vi "Read.vi"(8 "error in (no error)":errorcluster, 11 "UDP Reader in":refnum<class "UDP Reader.lvclass">) -> (0 "error out":errorcluster, 3 "UDP Reader out":refnum<class "UDP Reader.lvclass">)   [LabVIEW 2022 SP3, in "UDP Reader.lvlib" / "UDP Reader.lvclass"]
uses:
  UDP Reader.lvclass
  UDP Reader.lvclass/UDP Reader.ctl
  <vilib>/event_ctls.llb/usereventprio.ctl
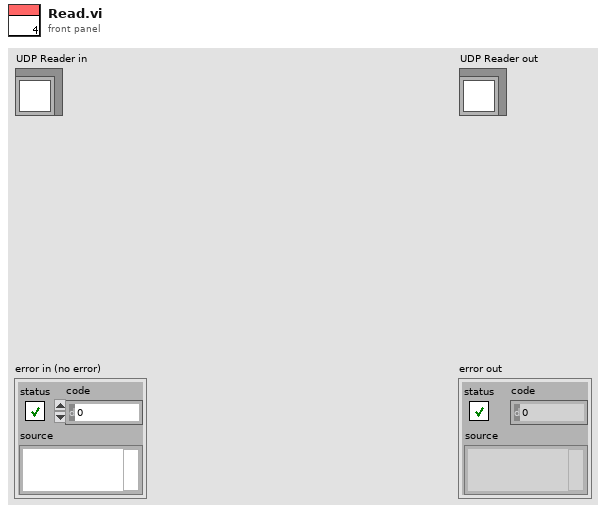
[diagram p1: front panel]
types:
  T1 = typedef "usereventprio.ctl" = enum32{"high priority", "normal priority"}
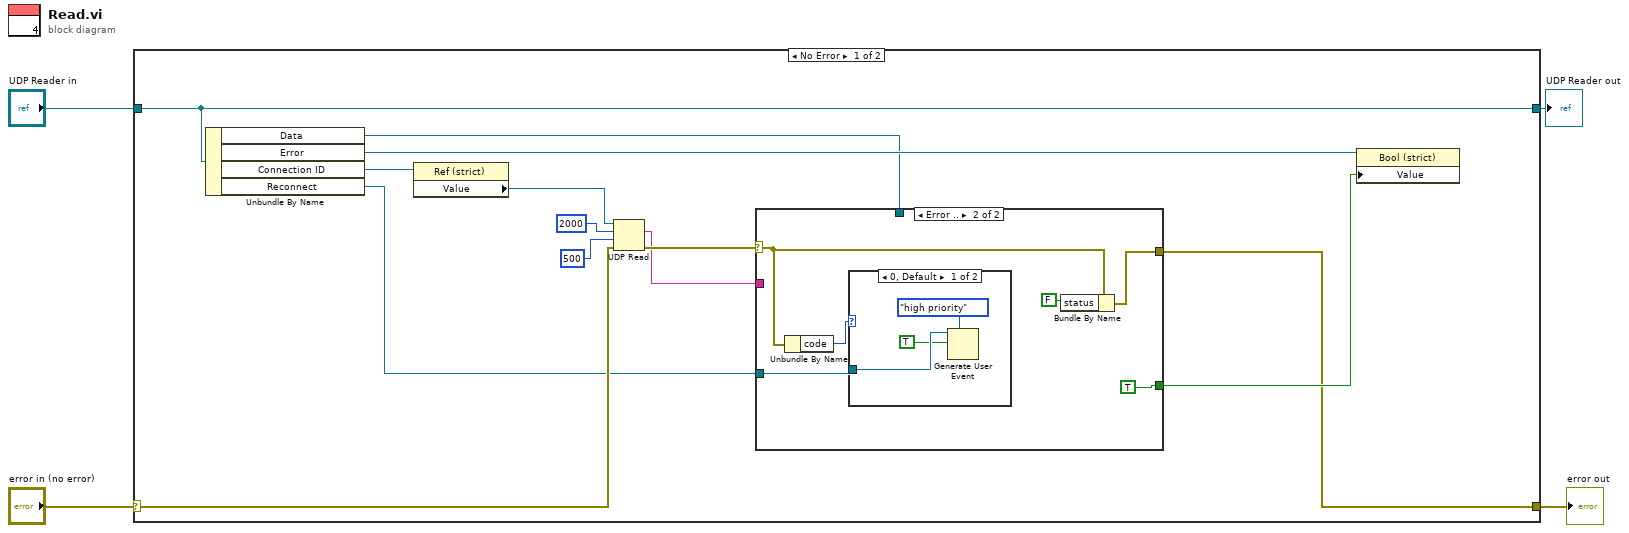
[diagram p0: block diagram]
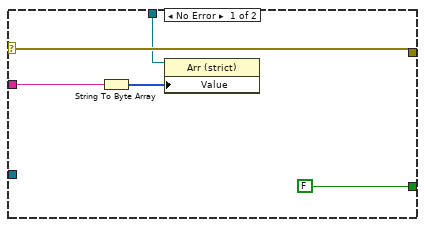
[diagram p2: hidden frame]
diagram:
  n1 = case shown="No Error" "error in (no error)" {
    selector: "error in (no error)" -> [w17 w33]
    tunnel: [w5 w33] -> w3
    tunnel: [w9 w32] -> w1
    tunnel: "UDP Reader in" -> [w9 w32]
    frame No Error {
      n2 = Unbundle By Name(w9) -> ("Data"=w6:refnum<vi>, "Error"=w8:refnum<vi>, "Connection ID"=w12:refnum<vi>, "Reconnect"=w10:refnum<user-event>)
      n3 = property class="Ref (strict)"(reference=w12) -> ("Value"=w11:refnum<k16>)  [unwired: 1 in, 2 out]
      n4 = UDP Read(connection ID=w11, max size (548)=2000, timeout ms (25000)=500, 8:w17) -> (data out=w13:string, error out=w14:errorcluster)  [unwired: 3 out]
      n5 = case shown="Error .." w14 {
        selector: w14 -> [w22 w24]
        tunnel: [w22 w23] -> w5
        tunnel: w13 -> [w21 _]
        tunnel: w10 -> [_ w26]
        tunnel: [FALSE ("data value") TRUE ("data value")] -> w7
        tunnel: w6 -> [w19 _]
        frame No Error {
          n6 = String To Byte Array(string=w21) -> (unsigned byte array=w18:u8[])
          n7 = property class="Arr (strict)"(reference=w19, "Value"=w18) -> ()  [unwired: 1 in, 2 out]
        }
        frame Error {
          n8 = Unbundle By Name(w24) -> ("code"=w28:i32)
          n9 = case shown="0, Default" w28 {
            tunnel: w26 -> [w31 _]
            frame 0, Default {
              n10 = Generate User Event(priority (normal)=usereventprio."high priority", user event=w31, event data cluster=TRUE ("event data")) -> ()  [unwired: 1 in, 2 out]
            }
            frame 56 {
            }
          }
          n11 = Bundle By Name(cluster=w24, "status"=FALSE) -> (w23:errorcluster)
        }
      }
      n12 = property class="Bool (strict)"(reference=w8, "Value"=w7) -> ()  [unwired: 1 in, 2 out]
    }
    frame Error {
    }
  }
  "error out" <- w3
  "UDP Reader out" <- w1
